vi "Untitled 1 (SubVI).vi"(0 "Boolean in":refnum<vi>, 1 "Stop Movement":bool, 2 "Go to Zero":bool, 3 "Position in":dbl, 4 "Automatic":bool, 6 "reference 3":refnum<vi>, 7 "Cycles Between Movements":i32, 8 "reference in":refnum<vi>, 9 "Go to 1":bool, 10 "Numeric":i32, 11 "Go to in":bool, 13 "Position 1":dbl) -> (14 "Indicator Pos 1":bool, 15 "Indicator Pos 2":bool)   [LabVIEW 2013, in "filenames.lvlib"]
uses:
  filenames.lvlib
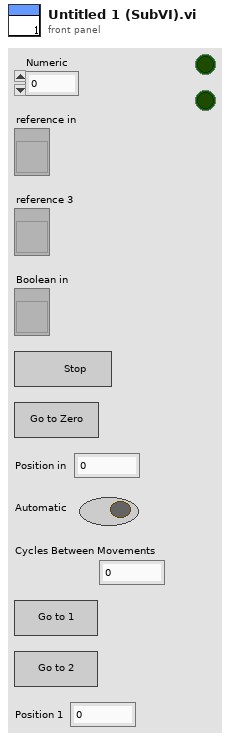
[diagram p1: front panel]
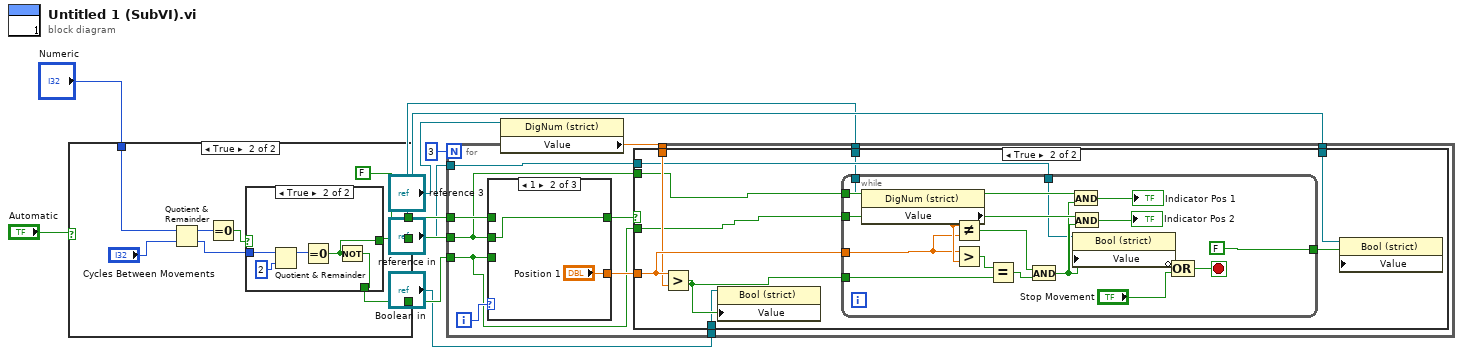
[diagram p0: block diagram]
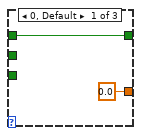
[diagram p3: hidden frame]
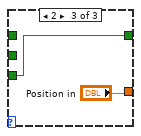
[diagram p4: hidden frame]
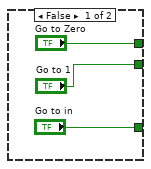
[diagram p5: hidden frame]
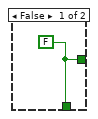
[diagram p6: hidden frame]
diagram:
  n1 = case shown="True" "Automatic" {
    tunnel: "Numeric" -> [_ w21]
    tunnel: ["Go to Zero" FALSE ("Go to Zero")] -> w7
    tunnel: ["Go to 1" w15] -> w8
    tunnel: ["Go to in" w16] -> w9
    frame False {
    }
    frame True {
      n2 = Quotient & Remainder(x=w21, y="Cycles Between Movements") -> (x-y*floor(x/y)=w19:i32, floor(x/y)=w17:i32)
      n3 = Equal To 0?(x=w19) -> (x = 0?=w18:bool)
      n4 = case shown="True" w18 {
        tunnel: w17 -> [_ w27]
        tunnel: [w22 w24] -> w16
        tunnel: [w22 w23] -> w15
        frame False {
          w22 = FALSE
        }
        frame True {
          n5 = Quotient & Remainder(x=w27, y=2) -> (x-y*floor(x/y)=w25:i32)  [unwired: 1 out]
          n6 = Equal To 0?(x=w25) -> (x = 0?=w23:bool)
          n7 = Not(x=w23) -> (.not. x?=w24:bool)
        }
      }
    }
  }
  n8 = property class="DigNum (strict)"(reference="reference 3") -> ("Value"=w5:dbl)  [unwired: 1 in, 2 out]
  n9 = for {
    N: 3 -> [_]
    tunnel: w7 -> [w37]
    tunnel: w8 -> [w33]
    tunnel: w9 -> [w32]
    tunnel: w5 -> [w34]
    tunnel: "Boolean in" -> [w31]
    tunnel: "reference in" -> [w30]
    tunnel: "reference 3" -> [w29]
    tunnel: "reference in" -> [w28]
    i -> [w38]
    n10 = case shown="1" w38 {
      tunnel: w37 -> [w66 _ _]
      tunnel: w33 -> [_ w68 _]
      tunnel: w32 -> [_ _ w70]
      tunnel: [w66 w68 w70] -> w36
      tunnel: [0.0 ("Position 2") "Position 1" "Position in"] -> w35
      frame 0, Default {
      }
      frame 1 {
      }
      frame 2 {
      }
    }
    n11 = case shown="True" w36 {
      tunnel: w35 -> [_ w48]
      tunnel: w34 -> [_ w47]
      tunnel: w33 -> [_ w44]
      tunnel: w32 -> [_ w45]
      tunnel: w31 -> [_ w42]
      tunnel: w30 -> [_ w41]
      tunnel: w29 -> [_ w40]
      tunnel: w28 -> [_ w39]
      frame False {
      }
      frame True {
        n12 = Greater?(x=w48, y=w47) -> (0:w46:bool)
        n13 = property class="Bool (strict)"(reference=w42, "Value"=w46) -> ()  [unwired: 1 in, 2 out]
        n14 = while {
          tunnel: w48 -> [w51]
          tunnel: w46 -> [w63]
          tunnel: w45 -> [w60]
          tunnel: w44 -> [w59]
          tunnel: [FALSE] -> w43
          tunnel: w41 -> [w50]
          tunnel: w40 -> [w49]
          stop <- w56 stop-if-true
          n15 = property class="DigNum (strict)"(reference=w49) -> ("Value"=w52:dbl)  [unwired: 1 in, 2 out]
          n16 = Not Equal?(x=w52, y=w51) -> (x != y?=w53:bool)
          n17 = Greater?(x=w51, y=w52) -> (0:w64:bool)
          n18 = Equal?(x=w64, y=w63) -> (x = y?=w58:bool)
          n19 = And(x=w53, y=w58) -> (x .and. y?=w54:bool)
          n20 = And(x=w59, y=w54) -> (x .and. y?=→"Indicator Pos 1":bool)
          n21 = And(x=w60, y=w54) -> (x .and. y?=→"Indicator Pos 2":bool)
          n22 = property class="Bool (strict)"(reference=w50, "Value"=w54) -> ()  [unwired: 1 in, 2 out]
          n23 = Compound Arithmetic op=OR(invert w54, "Stop Movement") -> (w56:bool)
        }
        n24 = property class="Bool (strict)"(reference=w39, "Value"=w43) -> ()  [unwired: 1 in, 2 out]
      }
    }
  }
